vi "Calculate z coord_v1.vi"(4 "Z factor":dbl[](array[numeric]), 6 "Z coord info":dbl[](array[numeric]), 7 "current (x,y)":dbl[](array[numeric]), 8 "xy grid min":dbl[](array[numeric]), 9 "index factor (DBL)":dbl, 10 "Za array":dbl[][](array[numeric]), 11 "Zp array":dbl[][](array[numeric])) -> (3 "cal z":dbl)   [LabVIEW 2010]
doc: "This VI computes the adaptive z coordinate value based on current (x,y) coordinate.\n\"Z coord info\" = [zp_eps, za_eps,zi]\nzp_eps: bound to posterior capsule\nza_eps: bound to anterior capsule\nzi: starting z coordinate of the trajectory"
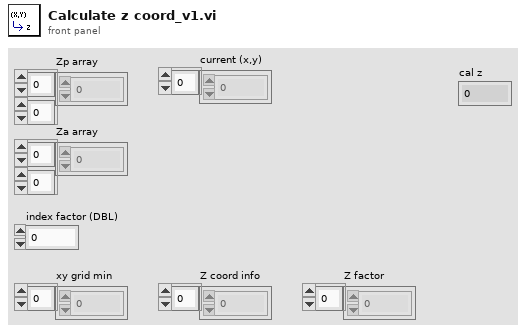
[diagram p1: front panel]
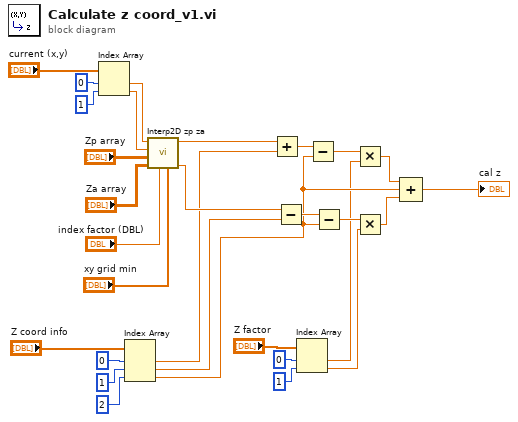
[diagram p0: block diagram]
diagram:
  n1 = Index Array(array="current (x,y)", index #1=0 ("index"), index #2=1 ("index")) -> (element #1=w25:dbl, element #2=w24:dbl)
  n2 = Index Array(array="Z coord info", index #1=0 ("index"), index #2=1 ("index"), index #3=2 ("index")) -> (element #1=w8:dbl, element #2=w7:dbl, element #3=w6:dbl)
  n3 = call "Interp2D zp za.vi"("xy grid min"="xy grid min", "index factor (DBL)"="index factor (DBL)", "Za array"="Za array", "Zp array"="Zp array", "current y"=w24, "current x"=w25) -> ("za"=w11:dbl, "zp"=w12:dbl)  [unwired: 4 in]
  n4 = Add(x=w12, y=w8) -> (x+y=w18:dbl)
  n5 = Subtract(x=w11, y=w7) -> (x-y=w19:dbl)
  n6 = Index Array(array="Z factor", index #1=0 ("index"), index #2=1 ("index")) -> (element #1=w2:dbl, element #2=w1:dbl)
  n7 = Subtract(x=w18, y=w6) -> (x-y=w15:dbl)
  n8 = Subtract(x=w19, y=w6) -> (x-y=w9:dbl)
  n9 = Multiply(x=w15, y=w2) -> (x*y=w16:dbl)
  n10 = Multiply(x=w9, y=w1) -> (x*y=w17:dbl)
  n11 = Compound Arithmetic op=ADD(w16, w6, w17) -> (→"cal z":dbl)
